vi "TableInterface.vi"(2 "Offset":u32, 3 "LastAddress":u32, 6 "START":bool, 7 "DDS/ARB":bool, 8 "CurrentAddress":u32, 9 "StopAddress":u32, 10 "StartAddress":u32, 11 "Increment":u32) -> (0 "One Wave Complete?":bool, 4 "NextAddress":u32, 5 "AddressRam":u32)   [LabVIEW 2018]
panel:
  # "When The pulse has been generated Once Completely, \ni.e All the memory has been scanned for once,\n then the signal will \nbe high, it is used to reset the trigger"
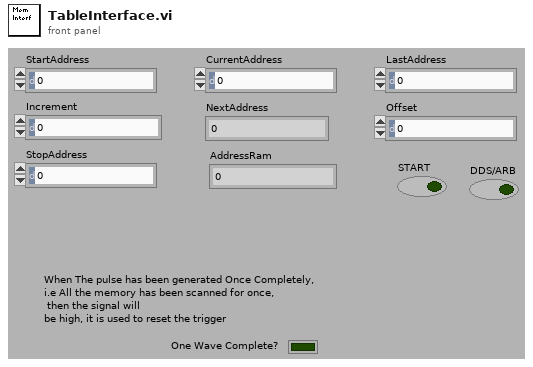
[diagram p1: front panel]
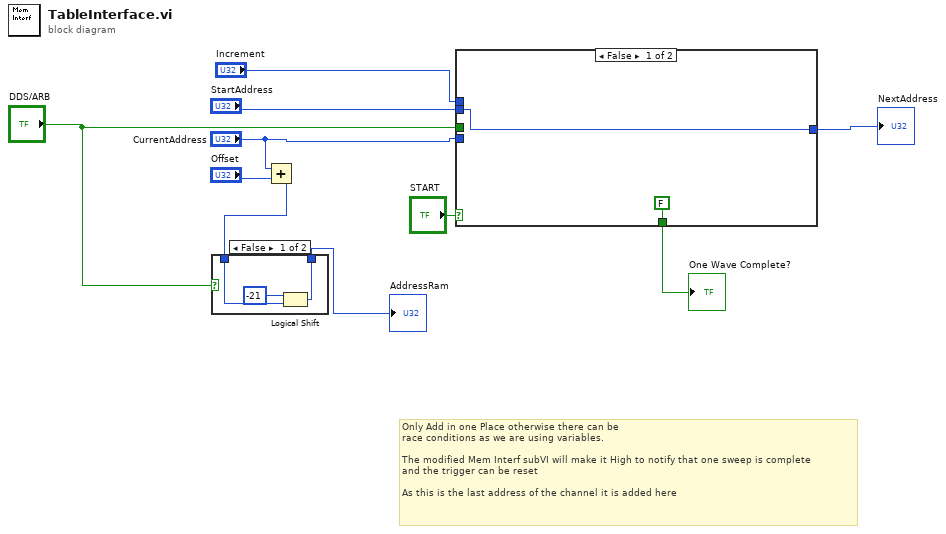
[diagram p0: block diagram]
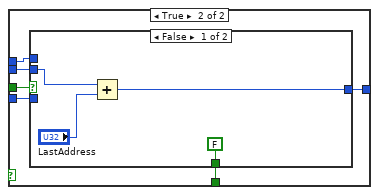
[diagram p2: hidden frame]
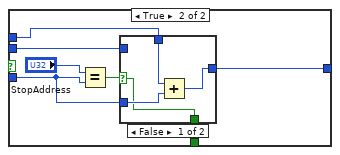
[diagram p3: hidden frame]
diagram:
  # "Only Add in one Place otherwise there can be \nrace conditions as we are using variables. \n\nThe modified Mem Interf subVI will make it High to notify that one sweep is complete \nand the trigger can be reset \n\nAs this is the last address of the channel it is added here"
  n1 = Add(x="CurrentAddress", y="Offset") -> (x+y=w2:u32)
  n2 = case shown="False" "DDS/ARB" {
    tunnel: [w12 w14] -> w10
    tunnel: w2 -> [w11 w14]
    frame False {
      n3 = Logical Shift(y=i8 -21, x=w11) -> (x << y=w12:u32)
    }
    frame True {
    }
  }
  "AddressRam" <- w10
  n4 = case shown="False" "START" {
    tunnel: "CurrentAddress" -> [_ w22]
    tunnel: [w16 w21] -> w5
    tunnel: "StartAddress" -> [w16 w20]
    tunnel: "Increment" -> [_ w19]
    tunnel: "DDS/ARB" -> [_ w18]
    tunnel: [FALSE w17] -> w1
    frame False {
    }
    frame True {
      n5 = case shown="False" w18 {
        tunnel: w19 -> [_ w29]
        tunnel: w22 -> [_ w31]
        tunnel: [w26 w32] -> w21
        tunnel: w20 -> [w24 w30]
        tunnel: [FALSE w27] -> w17
        frame False {
          n6 = Add(x=w24, y="LastAddress") -> (x+y=w26:u32)
        }
        frame True {
          n7 = Equal?(x="StopAddress", y=w31) -> (x = y?=w33:bool)
          n8 = case shown="False" w33 {
            selector: w33 -> [w34 w38]
            tunnel: [w36 w39] -> w32
            tunnel: w31 -> [w37 _]
            tunnel: w30 -> [_ w39]
            tunnel: w29 -> [w35 _]
            tunnel: [w34 w38] -> w27
            frame False {
              n9 = Add(x=w35, y=w37) -> (x+y=w36:u32)
            }
            frame True {
            }
          }
        }
      }
    }
  }
  "NextAddress" <- w5
  "One Wave Complete?" <- w1
